vi "Write.vi"(8 "error in (no error)":errorcluster, 10 "Value":T1, 11 "Double Float.lvclass_340760 in":refnum<class "Abs_U16 Integer.lvclass">) -> (0 "error out":errorcluster, 3 "Double Float.lvclass_340760 out":refnum<class "Abs_U16 Integer.lvclass">)   [LabVIEW 2021, in "Abs_U16 Integer.lvclass"]
uses:
  Abs_U16 Integer.lvclass
  Support/Type.ctl
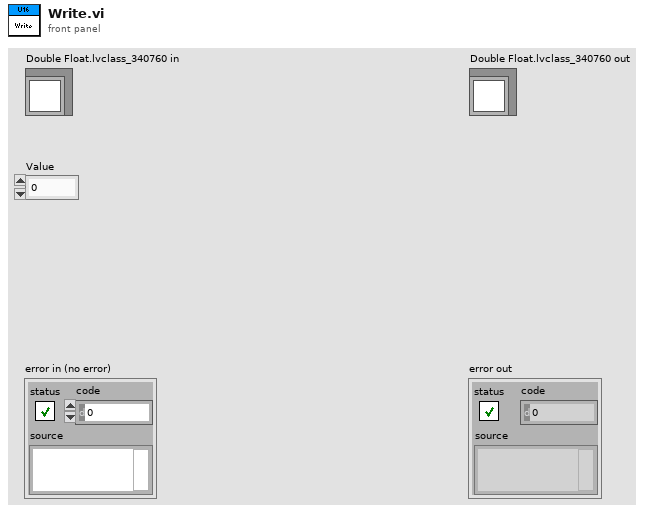
[diagram p1: front panel]
types:
  T1 = typedef "Abs_U16 Integer.lvclass/Type.ctl" = u16
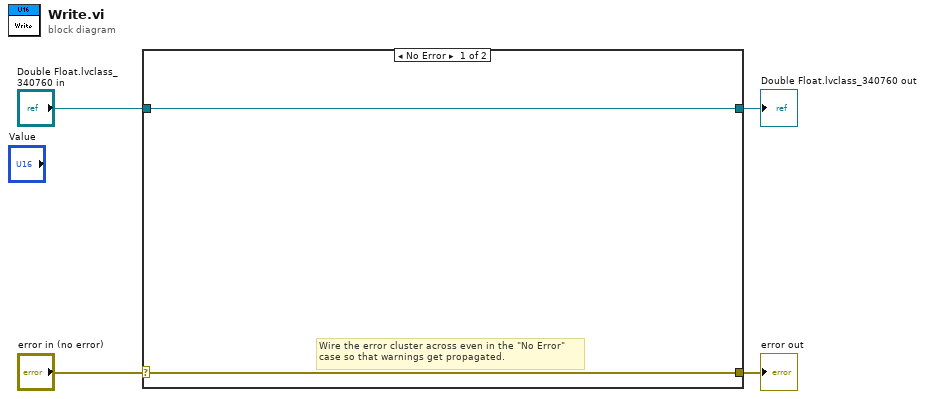
[diagram p0: block diagram]
diagram:
  n1 = case shown="No Error" "error in (no error)" {
    selector: "error in (no error)" -> [w5 w8]
    tunnel: [w5 w8] -> w3
    tunnel: [w6 w7] -> w1
    tunnel: "Double Float.lvclass_340760 in" -> [w6 w7]
    frame No Error {
      # "Wire the error cluster across even in the \"No Error\"\ncase so that warnings get propagated."
    }
    frame Error {
    }
  }
  "error out" <- w3
  "Double Float.lvclass_340760 out" <- w1
